vi "UMLEditor Main.vi"(1 "StartProject":string, 3 "StartTarget":string) -> ()   [LabVIEW 2012] (continued)
        n121 = call <resource>:"UMLEditor getDiagramInfo.vi"("localVariables"=w272, "error in (no error)"=w281) -> ("graph"=w279:refnum<class "Graph.lvclass">, "diagramType"=w275:T11, "error out"=w280:errorcluster)  [unwired: 15 out]
        n122 = event shown="[0] \"Picture\": Mouse Down" {
          selector: w273 -> [_ _ _ _ _ _ _ _ _ _ _ _ _ _ _ _ _ _ _ _ _ _ _ _ _ _ _ _ _ _ _ _ _ _ _ _ _ _ _ _ _ _ _ _ _ _ _ _ _ _ _ _ _ _ _ _ _]
          dyn-events: _ -> [_ _ _ _ _ _ _ _ _ _ _ _ _ _ _ _ _ _ _ _ _ _ _ _ _ _ _ _ _ _ _ _ _ _ _ _ _ _ _ _ _ _ _ _ _ _ _ _ _ _ _ _ _ _ _ _ _]
          timeout: 10 ("t") -> [_ _ _ _ _ _ _ _ _ _ _ _ _ _ _ _ _ _ _ _ _ _ _ _ _ _ _ _ _ _ _ _ _ _ _ _ _ _ _ _ _ _ _ _ _ _ _ _ _ _ _ _ _ _ _ _ _]
          tunnel: w283 -> [w289 _ _ _ _ _ _ _ _ _ w1719 _ _ _ _ _ _ _ _ _ _ _ _ _ _ _ _ _ _ _ _ _ _ _ _ _ _ _ _ _ _ _ _ _ _ _ _ _ _ _ _ _ _ _ _ _ _]
          tunnel: w277 -> [w284 w858 w1039 w1164 w1250 w1263 w1313 w1351 w1387 w1412 w1718 w2326 w2430 w2718 w2723 w2726 w3208 w3213 w3256 w3279 w3305 w3313 w3317 w3320 w3331 w3342 w3354 w3369 w3379 w3391 w3401 w3412 w3423 w3434 w3446 w3456 w3468 w3479 w3490 w3501 w3512 w3523 w3534 w3545 w3556 w3567 w3577 w3588 w3599 w3610 w3621 w3632 w3644 w3663 w3694 w3754 w3797]
          tunnel: [w295 w857 w1038 w1179 w1250 w1272 w1314 w1352 w1388 w1432 w1714 w2325 w2443 w2719 w2724 w2728 w3209 w3214 w3257 w3274 w3304 w3314 w3317 w3320 w3331 w3342 w3354 w3369 w3379 w3391 w3401 w3412 w3423 w3434 w3446 w3456 w3468 w3479 w3490 w3501 w3512 w3523 w3534 w3545 w3556 w3567 w3577 w3588 w3599 w3610 w3621 w3632 w3644 w3663 w3694 w3753 w3797] -> w278
          tunnel: w280 -> [w293 w862 w1042 w1185 w1251 w1262 w1312 w1350 w1386 w1428 w1717 w2324 w2439 w2715 w2721 w2732 w3207 w3215 w3249 w3276 w3306 w3315 w3319 w3324 w3333 w3344 w3356 w3373 w3384 w3395 w3406 w3417 w3428 w3439 w3450 w3461 w3472 w3483 w3494 w3505 w3516 w3527 w3538 w3549 w3560 w3571 w3582 w3589 w3600 w3611 w3622 w3633 w3646 w3656 w3692 w3750 w3802]
          tunnel: [w292 w864 w1044 w1174 w1251 w1262 w1312 w1350 w1386 w1423 w1716 w2323 w2440 w2715 w2721 w2731 w3207 w3215 w3249 w3260 w3306 w3315 w3319 w3323 w3332 w3343 w3355 w3372 w3383 w3394 w3405 w3416 w3427 w3438 w3449 w3460 w3471 w3482 w3493 w3504 w3515 w3526 w3537 w3548 w3559 w3570 w3581 w3590 w3601 w3612 w3623 w3634 w3645 w3657 w3695 w3755 w3801] -> w282
          tunnel: w279 -> [w296 w855 w1036 w1170 _ _ _ _ _ w1424 w1715 _ w2438 _ _ w2730 _ _ _ _ _ _ _ _ _ _ _ _ _ _ _ _ _ _ _ _ _ _ _ _ _ _ _ _ _ _ _ _ _ _ _ _ _ _ _ w3752 _]
          tunnel: w275 -> [w294 _ _ _ _ _ _ _ _ _ _ _ w2437 _ _ w2729 _ _ _ _ _ _ _ _ _ _ w3350 _ _ _ _ _ _ _ _ _ _ _ _ _ _ _ _ _ _ _ _ _ _ _ _ _ _ _ _ _ _]
          tunnel: w272 -> [_ w854 _ _ _ _ _ _ _ _ _ _ _ _ _ w2727 _ _ _ _ _ _ _ _ _ _ _ _ _ _ _ _ _ _ _ _ _ _ _ _ _ _ _ _ _ _ _ _ _ _ _ _ _ _ _ _ _]
          tunnel: w271 -> [w285 _ _ _ _ _ _ _ _ w1401 w1713 _ _ _ _ _ _ _ _ _ _ w3307 w3316 _ _ _ _ _ _ _ _ _ _ _ _ _ _ _ _ _ _ _ _ _ _ _ _ _ _ _ _ _ _ _ _ _ _]
          event "Picture": Mouse Down {
            # "Shift"
            n123 = event-data() -> ("Source"=w297:T41, "Button"=w291:u16, "Mods.Double Click"=w288:bool, "PlatMods.Ctrl"=w287:bool, "PlatMods.Shift"=w286:bool)  [unwired: 1 out]
            n124 = case shown="1, Default" w291 {
              tunnel: w297 -> [_ _]
              tunnel: w296 -> [w304 _]
              tunnel: [w339 w851] -> w295
              tunnel: w294 -> [w338 _]
              tunnel: w293 -> [w331 w850]
              tunnel: w284 -> [w324 w851]
              tunnel: [w326 w850] -> w292
              tunnel: w291 -> [w325 _]
              tunnel: w288 -> [w314 _]
              tunnel: w287 -> [w313 _]
              tunnel: w289 -> [_ _]
              tunnel: w286 -> [w303 _]
              tunnel: w285 -> [w299 _]
              frame 1, Default {
                n125 = property on="Picture" class="Pict"() -> ("Mouse"=w318:T42, "Draw Area Size"=w317:T43, "Origin"=w315:T44)  [unwired: 2 in, 2 out]
                n126 = Unbundle By Name(w324) -> ("graphics"=w307:refnum<class "Graphics.lvclass">, "SelectedNodes"=w320:refnum<class "AbstractNode.lvclass">[])
                n127 = Unbundle By Name(w324) -> ("HotSpotNode"=w300:refnum<class "AbstractNode.lvclass">, "HotSpotCursor"=w301:bool, "HotSpotFunction"=w302:T19, "zoom"=w327:dbl, "offset"=w329:T12)
                n128 = Unbundle By Name(w318) -> ("Mouse Position"=w330:cluster{"X":i32, "Y":i32})
                n129 = call <resource>:"UMLEditor ToolBarSettings.vi"("localVariables"=w324, "error in (no error)"=w331) -> ("toolType"=w337:T9, "tools"=w336:T10, "prototypeEdge"=w335:refnum<class "AbstractEdge.lvclass">, "prototypeNode"=w334:refnum<class "AbstractNode.lvclass">, "error out"=w312:errorcluster)  [unwired: 2 in, 11 out]
                n130 = Array Size(array=w320) -> (size(s)=w322:i32)
                n131 = Tick Count (ms)() -> (millisecond timer value=w319:u32)
                n132 = Greater?(x=w322, y=1) -> (0:w323:bool)
                n133 = Add(x=w329, y=w330) -> (x+y=w328:T12)
                n134 = call <resource>:"UMLEditor IsMouseOutsideDrawingArea.vi"("Mouse"=w318, "Draw Area Size"=w317, "Origin"=w315) -> ("OutsideDrawingArea"=w316:bool)  [unwired: 2 in, 14 out]
                n135 = Divide(x=w328, y=w327) -> (x/y=w311:T12)
                n136 = Bundle By Name(cluster=w324, "state"=UMLEditor_statesType."Repaint", "lastMousePoint"=w311) -> (w333:T7)
                n137 = call <resource>:"UMLEditor_FindObject.vi"("offset"=w311, "error in"=w312, "graphics"=w307, "graph"=w304) -> ("error out"=w310:errorcluster, "NodeFound"=w309:bool, "node"=w308:refnum<class "AbstractNode.lvclass">, "edge"=w306:refnum<class "AbstractEdge.lvclass">, "EdgeFound"=w305:bool)  [unwired: 2 in, 1 out]
                n138 = case shown="False" w316 {
                  tunnel: w310 -> [w372 w849]
                  tunnel: w309 -> [w345 _]
                  tunnel: w305 -> [w354 _]
                  tunnel: w306 -> [w371 _]
                  tunnel: w308 -> [w370 _]
                  tunnel: [w369 w847] -> w339
                  tunnel: w338 -> [w367 _]
                  tunnel: w337 -> [w366 _]
                  tunnel: w336 -> [w365 _]
                  tunnel: w335 -> [w364 _]
                  tunnel: w334 -> [w363 _]
                  tunnel: w304 -> [w362 _]
                  tunnel: w333 -> [w361 w848]
                  tunnel: w311 -> [w360 _]
                  tunnel: [w359 w849] -> w326
                  tunnel: w325 -> [w358 _]
                  tunnel: w323 -> [w357 _]
                  tunnel: w320 -> [w356 _]
                  tunnel: w319 -> [_ _]
                  tunnel: w317 -> [_ _]
                  tunnel: w314 -> [w346 _]
                  tunnel: w313 -> [w351 _]
                  tunnel: w307 -> [w349 _]
                  tunnel: w303 -> [w344 _]
                  tunnel: w302 -> [_ _]
                  tunnel: w301 -> [w342 _]
                  tunnel: w300 -> [w341 _]
                  tunnel: w299 -> [w340 _]
                  frame False {
                    n139 = Or(x=w345, y=w354) -> (x .or. y?=w353:bool)
                    n140 = And(x=w345, y=w344) -> (x .and. y?=w343:bool)
                    n141 = Compound Arithmetic op=AND(w346, w353) -> (w355:bool)
                    n142 = case shown="False" w355 {
                      tunnel: w372 -> [w392 w798]
                      tunnel: [w391 w797] -> w359
                      tunnel: w345 -> [w394 w796]
                      tunnel: w354 -> [w382 w791]
                      tunnel: w366 -> [w381 _]
                      tunnel: w361 -> [w397 w795]
                      tunnel: [w396 w794] -> w368
                      tunnel: w371 -> [w395 w793]
                      tunnel: w370 -> [w393 w792]
                      tunnel: w360 -> [w390 w789]
                      tunnel: w365 -> [w389 _]
                      tunnel: w367 -> [w388 _]
                      tunnel: w364 -> [w387 _]
                      tunnel: w363 -> [w386 _]
                      tunnel: w362 -> [w385 _]
                      tunnel: w358 -> [_ _]
                      tunnel: w357 -> [w384 _]
                      tunnel: w356 -> [w383 _]
                      tunnel: UMLEditor_tooltype."None" ("t") -> [w380 _]
                      tunnel: w351 -> [w377 w790]
                      tunnel: [TRUE ("butDwn") w788] -> w350
                      tunnel: w349 -> [w378 _]
                      tunnel: w343 -> [w376 _]
                      tunnel: [w376 w788] -> w348
                      tunnel: [w377 w788] -> w347
                      tunnel: w346 -> [_ _]
                      tunnel: w342 -> [w375 _]
                      tunnel: w341 -> [w374 _]
                      tunnel: w340 -> [w373 _]
                      frame False {
                        # "Single Click"
                        n143 = case shown="False" w376 {
                          tunnel: w397 -> [w420 w776]
                          tunnel: [w419 w775] -> w396
                          tunnel: w395 -> [w418 _]
                          tunnel: w394 -> [w417 _]
                          tunnel: w393 -> [w416 w772]
                          tunnel: w392 -> [w415 w771]
                          tunnel: [w414 w771] -> w391
                          tunnel: w390 -> [w413 w774]
                          tunnel: w389 -> [w412 _]
                          tunnel: w388 -> [w411 _]
                          tunnel: w387 -> [w410 _]
                          tunnel: w386 -> [w409 _]
                          tunnel: w385 -> [w408 _]
                          tunnel: w384 -> [w407 _]
                          tunnel: w383 -> [w406 w773]
                          tunnel: w382 -> [w405 _]
                          tunnel: w381 -> [w404 _]
                          tunnel: w380 -> [w402 _]
                          tunnel: w378 -> [w401 _]
                          tunnel: [_ w769] -> _
                          tunnel: w375 -> [w400 _]
                          tunnel: w374 -> [w399 _]
                          tunnel: w373 -> [w398 _]
                          frame False {
                            n144 = Select(t=w402, s=w405, f=w404) -> (s? t:f=w403:T9)
                            n145 = case shown="False" w400 {
                              tunnel: w420 -> [w440 w761]
                              tunnel: [w439 w760] -> w419
                              tunnel: w418 -> [w438 _]
                              tunnel: w417 -> [w437 _]
                              tunnel: w416 -> [w436 _]
                              tunnel: w415 -> [w435 w763]
                              tunnel: [w434 w762] -> w414
                              tunnel: w413 -> [w433 w759]
                              tunnel: w412 -> [w432 _]
                              tunnel: w411 -> [w431 _]
                              tunnel: w410 -> [w430 _]
                              tunnel: w409 -> [w429 _]
                              tunnel: w408 -> [w428 _]
                              tunnel: w407 -> [w427 _]
                              tunnel: w406 -> [w426 _]
                              tunnel: w405 -> [w425 _]
                              tunnel: w403 -> [w424 _]
                              tunnel: w401 -> [w423 _]
                              tunnel: w400 -> [w422 _]
                              tunnel: w399 -> [_ w758]
                              tunnel: w398 -> [w421 _]
                              frame False {
                                n146 = case shown="\"Node\"" w424 {
                                tunnel: w425 -> [w455 _ _]
                                tunnel: w440 -> [w454 w591 w640]
                                tunnel: [w453 w590 w639] -> w439
                                tunnel: w438 -> [w452 _ _]
                                tunnel: w437 -> [w451 w586 w637]
                                tunnel: w436 -> [w450 w585 w636]
                                tunnel: w435 -> [w449 w583 w635]
                                tunnel: [w448 w587 w634] -> w434
                                tunnel: w433 -> [w447 w582 w638]
                                tunnel: w432 -> [_ _ w633]
                                tunnel: w431 -> [_ _ w632]
                                tunnel: w430 -> [_ _ _]
                                tunnel: w429 -> [_ w594 _]
                                tunnel: w428 -> [w446 w584 w631]
                                tunnel: w427 -> [w445 _ _]
                                tunnel: w426 -> [w444 _ _]
                                tunnel: w423 -> [w443 _ _]
                                tunnel: w422 -> [w442 _ _]
                                tunnel: w421 -> [w441 _ _]
                                frame "None", Default {
                                # "Select"
                                n147 = case shown="False" w455 {
                                tunnel: w454 -> [w465 w560]
                                tunnel: [w464 w559] -> w453
                                tunnel: w452 -> [_ w523]
                                tunnel: w451 -> [w466 _]
                                tunnel: w450 -> [w463 _]
                                tunnel: w449 -> [w462 w539]
                                tunnel: [w461 w539] -> w448
                                tunnel: w447 -> [w460 w534]
                                tunnel: w446 -> [_ _]
                                tunnel: w445 -> [w459 _]
                                tunnel: w444 -> [w458 _]
                                tunnel: w443 -> [_ w520]
                                tunnel: w442 -> [w457 _]
                                tunnel: w441 -> [w456 _]
                                frame False {
                                n148 = case shown="True" w466 {
                                tunnel: w465 -> [w471 w518]
                                tunnel: [w476 w517] -> w464
                                tunnel: w463 -> [w477 _]
                                tunnel: w462 -> [w478 w514]
                                tunnel: [w475 w514] -> w461
                                tunnel: w460 -> [w474 w511]
                                tunnel: w459 -> [w473 _]
                                tunnel: w458 -> [w472 _]
                                tunnel: w457 -> [w468 _]
                                tunnel: w456 -> [w467 _]
                                frame True {
                                # "Node Selected"
                                n149 = case shown="False" w468 {
                                tunnel: w467 -> [w479 _]
                                frame False {
                                n150 = call-poly <vilib>:"Set Cursor.vi"("VI reference (current VI)"=w479, "icon"=u16 5) -> ()  [unwired: 1 in, 9 out]
                                }
                                frame True {
                                }
                                }
                                n151 = Bundle By Name(cluster=w471, "state"=UMLEditor_statesType."Idle") -> (w469:T7)
                                n152 = case shown="True" w473 {
                                tunnel: w478 -> [w490 w494]
                                tunnel: w477 -> [w489 w493]
                                tunnel: w469 -> [w486 w492]
                                tunnel: [w485 w498] -> w476
                                tunnel: [w483 w494] -> w475
                                tunnel: w474 -> [w481 w497]
                                tunnel: w472 -> [_ w496]
                                frame False {
                                n153 = call-dynamic "getBounds.vi"("reference"=w489, "error in (no error)"=w490) -> ("reference out"=w488:refnum<class "AbstractNode.lvclass">, "bounds"=w487:T13, "error out"=w483:errorcluster)  [unwired: 15 in]
                                n154 = Build Array(w488) -> (w482:refnum<class "AbstractNode.lvclass">[])
                                n155 = Bundle By Name(cluster=w486, "selcted"=UMLEditor_tooltype."Node", "SelectedNodes"=w482, "dragStartBounds"=w487, "dragStartPoint"=w481, "newSelected"=TRUE, "lastMousePoint"=w481) -> (w485:T7)
                                }
                                frame True {
                                # "If many nodes allready selected move these"
                                n156 = Search 1D Array(1D array=w496, element=w493) -> (index of element=w495:i32)  [unwired: 1 out]
                                n157 = case shown="Default" w495 {
                                tunnel: w492 -> [w503 w510]
                                tunnel: [w502 w509] -> w498
                                tunnel: w497 -> [w501 w508]
                                tunnel: w493 -> [_ w505]
                                frame Default {
                                n158 = Bundle By Name(cluster=w503, "selcted"=UMLEditor_tooltype."Node", "dragStartPoint"=w501, "newSelected"=TRUE, "lastMousePoint"=w501) -> (w502:T7)
                                }
                                frame -1 {
                                n159 = Build Array(w505) -> (w504:refnum<class "AbstractNode.lvclass">[])
                                n160 = Bundle By Name(cluster=w510, "selcted"=UMLEditor_tooltype."Node", "dragStartPoint"=w508, "newSelected"=TRUE, "lastMousePoint"=w508, "SelectedNodes"=w504) -> (w509:T7)
                                }
                                }
                                }
                                }
                                }
                                frame False {
                                # "None Selected\nArea Select???"
                                n161 = Bundle By Name(cluster=w518, "selcted"=UMLEditor_tooltype."None", "SelectedNodes"=refnum<class "AbstractNode.lvclass">[] [], "dragStartBounds"=T13 {"x"=0.0, "y"=0.0, "width"=0.0, "height"=0.0}, "dragStartPoint"=w511, "rubberBandStart"=w511, "newSelected"=TRUE, "state"=UMLEditor_statesType."Idle", "lastMousePoint"=w511) -> (w517:T7)
                                }
                                }
                                }
                                frame True {
                                w556 = 25.0 ("y")
                                n162 = To More Specific Class(target class=refnum<class "GeneralPathEdge.lvclass"> refnum ("reference"), reference=w523) -> (specific class reference=w521:refnum<class "GeneralPathEdge.lvclass">)  [unwired: 1 in, 1 out]
                                n163 = call-dynamic "getPoints.vi"("reference"=w521, "error in (no error)"=w539) -> ("reference out"=w537:refnum<class "GeneralPathEdge.lvclass">, "points"=w535:T12[], "error out"=w538:errorcluster)  [unwired: 15 in]
                                n164 = Array Size(array=w535) -> (size(s)=w536:i32)
                                n165 = case shown="4" w536 {
                                tunnel: w535 -> [_ w569]
                                tunnel: w534 -> [_ w564]
                                tunnel: [_ w561] -> w529
                                frame Default {
                                }
                                frame 4 {
                                # "Egde selected"
                                n166 = Index Array(array=w569, index #1=1 ("index")) -> (element #1=w567:T12, element #2=w566:T12)  [unwired: 1 in]
                                n167 = Build Array(w567, w566) -> (w565:T12[])
                                n168 = call <resource>:"Point getDistanceToLine.vi"("point1"=w564, "line"=w565) -> ("minDistance"=w563:dbl)  [unwired: 1 in, 16 out]
                                n169 = Less?(x=w563, y=25.0) -> (x < y?=w561:bool)
                                }
                                }
                                n170 = Index Array(array=w535) -> (element=w555:T12)  [unwired: 1 in]
                                n171 = Delete From Array(array=w535) -> (deleted portion=w554:T12)  [unwired: 2 in, 1 out]
                                n172 = call-dynamic "GetTextPositions.vi"("reference"=w537, "GraphicsRef"=w520, "error in (no error)"=w538) -> ("reference out"=w547:refnum<class "GeneralPathEdge.lvclass">, "connectionPoints"=w546:T12[], "error out"=w548:errorcluster)  [unwired: 14 in]
                                n173 = Index Array(array=w546) -> (element=w545:T12)  [unwired: 1 in]
                                n174 = call <resource>:"Point getDistance.vi"("point1"=w555, "point2"=w534) -> ("distance"=w558:dbl)  [unwired: 1 in, 16 out]
                                n175 = call <resource>:"Point getDistance.vi"("point1"=w554, "point2"=w534) -> ("distance"=w557:dbl)  [unwired: 1 in, 16 out]
                                n176 = call-dynamic "getEnd.vi"("reference"=w547, "error in (no error)"=w548) -> ("reference out"=w552:refnum<class "GeneralPathEdge.lvclass">, "endNode"=w526:refnum<class "AbstractNode.lvclass">, "error out"=w553:errorcluster)  [unwired: 14 in, 1 out]
                                n177 = call <resource>:"Point getDistance.vi"("point1"=w545, "point2"=w534) -> ("distance"=w544:dbl)  [unwired: 1 in, 16 out]
                                n178 = Less?(x=w557, y=w556) -> (x < y?=w532:bool)
                                n179 = Less?(x=w558, y=w556) -> (x < y?=w531:bool)
                                n180 = Less?(x=w544, y=40.0) -> (x < y?=w533:bool)
                                n181 = call-dynamic "getStart.vi"("reference"=w552, "error in (no error)"=w553) -> ("startNode"=w525:refnum<class "AbstractNode.lvclass">, "error out"=w551:errorcluster)  [unwired: 14 in, 2 out]
                                n182 = Select(t=w526, s=w532, f=w525) -> (s? t:f=w542:refnum<class "AbstractNode.lvclass">)
                                n183 = Unbundle By Name(w551) -> ("status"=w550:bool)
                                n184 = Build Array(w526, w525) -> (w524:refnum<class "AbstractNode.lvclass">[])
                                n185 = Compound Arithmetic op=OR(w529, w531, w532, w533) -> (w530:bool)
                                n186 = Build Array(w542) -> (w528:refnum<class "AbstractNode.lvclass">[])
                                n187 = Compound Arithmetic op=AND(w530, invert w550) -> (w549:bool)
                                n188 = Select(t=w524, s=w529, f=w528) -> (s? t:f=w527:refnum<class "AbstractNode.lvclass">[])
                                n189 = Select(t=refnum<class "AbstractNode.lvclass">[] [], s=w533, f=w527) -> (s? t:f=w540:refnum<class "AbstractNode.lvclass">[])
                                n190 = case shown="True" w549 {
                                tunnel: w560 -> [w576 w581]
                                tunnel: [w575 w580] -> w559
                                tunnel: w523 -> [w572 w577]
                                tunnel: w534 -> [w571 _]
                                tunnel: w540 -> [w570 _]
                                frame True {
                                n191 = Bundle By Name(cluster=w576, "selcted"=UMLEditor_tooltype."Edge", "selectedEdge"=w572, "dragStartPoint"=w571, "newSelected"=TRUE, "SelectedNodes"=w570) -> (w575:T7)
                                }
                                frame False {
                                n192 = Bundle By Name(cluster=w581, "selcted"=UMLEditor_tooltype."Edge", "selectedEdge"=w577, "newSelected"=TRUE) -> (w580:T7)
                                }
                                }
                                }
                                }
                                }
                                frame "Node" {
                                # "Node Tool"
                                n193 = call-dynamic "clone.vi"("reference"=w594, "error in (no error)"=w583) -> ("clonedAbstractNode"=w588:refnum<class "AbstractNode.lvclass">, "error out"=w593:errorcluster)  [unwired: 15 in, 1 out]
                                n194 = call-dynamic "add.vi"("reference"=w584, "node"=w588, "point"=w582, "error in (no error)"=w593) -> ("added"=w592:bool, "error out"=w589:errorcluster)  [unwired: 13 in, 1 out]
                                n195 = case shown="False" w592 {
                                tunnel: w591 -> [w602 w622]
                                tunnel: [w601 w620] -> w590
                                tunnel: w589 -> [w597 w630]
                                tunnel: w588 -> [w595 w629]
                                tunnel: w582 -> [w599 w618]
                                tunnel: [w598 w623] -> w587
                                tunnel: w586 -> [w603 _]
                                tunnel: w585 -> [w600 _]
                                frame False {
                                n196 = call-dynamic "Destroy.vi"("reference"=w595, "error in (no error)"=w597) -> ("error out"=w596:errorcluster)  [unwired: 16 in, 1 out]
                                n197 = case shown="False" w603 {
                                tunnel: w602 -> [w605 w614]
                                tunnel: [w605 w613] -> w601
                                tunnel: w596 -> [w604 w616]
                                tunnel: w600 -> [_ w608]
                                tunnel: w599 -> [_ w610]
                                tunnel: [w604 w612] -> w598
                                frame False {
                                }
                                frame True {
                                # "Node Found"
                                n198 = call-dynamic "getBounds.vi"("reference"=w608, "error in (no error)"=w616) -> ("bounds"=w615:T13, "error out"=w612:errorcluster)  [unwired: 15 in, 1 out]
                                n199 = Build Array(w608) -> (w611:refnum<class "AbstractNode.lvclass">[])
                                n200 = Bundle By Name(cluster=w614, "selcted"=UMLEditor_tooltype."Node", "SelectedNodes"=w611, "dragStartBounds"=w615, "dragStartPoint"=w610, "lastMousePoint"=w610, "newSelected"=TRUE, "toolType"=UMLEditor_tooltype."None", "tool"=UMLEditor_toolsType."CD_Select") -> (w613:T7)
                                n201 = call <resource>:"UMLEditor UpdatesToolbuttons.vi"() -> ()  [unwired: 6 in, 14 out]
                                }
                                }
                                }
                                frame True {
                                # "Added"
                                n202 = call-dynamic "getBounds.vi"("reference"=w629, "error in (no error)"=w630) -> ("reference out"=w627:refnum<class "AbstractNode.lvclass">, "bounds"=w628:T13, "error out"=w624:errorcluster)  [unwired: 15 in]
                                n203 = Build Array(w627) -> (w619:refnum<class "AbstractNode.lvclass">[])
                                n204 = Bundle By Name(cluster=w622, "selcted"=UMLEditor_tooltype."Node", "SelectedNodes"=w619, "dragStartBounds"=w628, "dragStartPoint"=w618, "lastMousePoint"=w618) -> (w621:T7)
                                n205 = call <resource>:"UMLEditor setDiagramInfo.vi"("error in (no error)"=w624, "localVariablesIn"=w621, "action"=enum16{"Name/Dir", "Unsaved", "Saved"}."Unsaved") -> ("localVariablesOut"=w620:T7, "error out"=w623:errorcluster)  [unwired: 2 in, 13 out]
                                }
                                }
                                }
                                frame "Edge" {
                                # "Edge Tool"
                                n206 = case shown="True" w637 {
                                tunnel: w640 -> [w642 w655]
                                tunnel: [w641 w654] -> w639
                                tunnel: w638 -> [_ w653]
                                tunnel: w636 -> [_ w652]
                                tunnel: w635 -> [w645 w651]
                                tunnel: [w645 w649] -> w634
                                tunnel: w633 -> [_ w648]
                                tunnel: w632 -> [_ w647]
                                tunnel: w631 -> [_ w646]
                                frame False {
                                n207 = call <resource>:"UMLEditor UpdatesToolbuttons.vi"() -> ()  [unwired: 6 in, 14 out]
                                n208 = Bundle By Name(cluster=w642, "toolType"=UMLEditor_tooltype."None", "tool"=UMLEditor_toolsType."CD_Select") -> (w641:T7)
                                }
                                frame True {
                                n209 = case shown="\"Class\"" w647 {
                                tunnel: w652 -> [_ w685 w698 w711 w743]
                                tunnel: w651 -> [w656 w684 w699 w712 w742]
                                tunnel: [TRUE w668 w695 w707 w727] -> w650
                                tunnel: [w656 w667 w697 w710 w734] -> w649
                                tunnel: w648 -> [_ w665 w686 w706 w720]
                                tunnel: w646 -> [_ _ _ _ w736]
                                frame "None", Default {
                                }
                                frame "Class" {
                                w664 = UMLEditor_toolsType."CD_Dependency" ("tools")
                                n210 = call <resource>:"AbstractNode_GetObjectStatus.vi"("reference in"=w685, "error in (no error)"=w684) -> ("Class name"=w659:string, "error out"=w667:errorcluster)  [unwired: 16 out]
                                n211 = Match Pattern(string=w659, regular expression="NoteNode$") -> (offset past match=w680:i32)  [unwired: 4 out]
                                n212 = Match Pattern(string=w659, regular expression="InterfaceNode$") -> (offset past match=w679:i32)  [unwired: 4 out]
                                n213 = Match Pattern(string=w659, regular expression="ClassNode$") -> (offset past match=w678:i32)  [unwired: 4 out]
                                n214 = Match Pattern(string=w659, regular expression="PackageNode$") -> (offset past match=w661:i32)  [unwired: 4 out]
                                n215 = Equal?(x=w665, y=UMLEditor_toolsType."CD_NoteConn" ("tools")) -> (x = y?=w672:bool)
                                n216 = In Range and Coerce(upper limit=UMLEditor_toolsType."CD_Composite" ("tools"), x=w665, lower limit=w664) -> (In Range?=w675:bool)  [unwired: 1 out]
                                n217 = Equal?(x=w664, y=w665) -> (x = y?=w662:bool)
                                n218 = Greater Or Equal To 0?(x=w680) -> (x >= 0?=w671:bool)
                                n219 = Greater Or Equal To 0?(x=w679) -> (x >= 0?=w677:bool)
                                n220 = Greater Or Equal To 0?(x=w678) -> (x >= 0?=w676:bool)
                                n221 = Greater Or Equal To 0?(x=w661) -> (x >= 0?=w658:bool)
                                n222 = And(x=w672, y=w671) -> (x .and. y?=w669:bool)
                                n223 = Or(x=w677, y=w676) -> (x .or. y?=w674:bool)
                                n224 = And(x=w675, y=w674) -> (x .and. y?=w670:bool)
                                n225 = And(x=w662, y=w658) -> (x .and. y?=w663:bool)
                                n226 = Compound Arithmetic op=OR(w670, w669, w663) -> (w668:bool)
                                }
                                frame "Sequency" {
                                n227 = call <resource>:"AbstractNode_GetObjectStatus.vi"("reference in"=w698, "error in (no error)"=w699) -> ("Class name"=w688:string, "error out"=w697:errorcluster)  [unwired: 16 out]
                                n228 = Match Pattern(string=w688, regular expression="CallNode$") -> (offset past match=w690:i32)  [unwired: 4 out]
                                n229 = Match Pattern(string=w688, regular expression="NoteNode$") -> (offset past match=w702:i32)  [unwired: 4 out]
                                n230 = Equal?(x=w686, y=UMLEditor_toolsType."SQD_Call" ("tools")) -> (x = y?=w691:bool)
                                n231 = Equal?(x=w686, y=UMLEditor_toolsType."SQD_NoteConn" ("tools")) -> (x = y?=w701:bool)
                                n232 = Greater Or Equal To 0?(x=w690) -> (x >= 0?=w692:bool)
                                n233 = Greater Or Equal To 0?(x=w702) -> (x >= 0?=w700:bool)
                                n234 = And(x=w691, y=w692) -> (x .and. y?=w687:bool)
                                n235 = And(x=w701, y=w700) -> (x .and. y?=w696:bool)
                                n236 = Compound Arithmetic op=OR(w687, w696) -> (w695:bool)
                                }
                                frame "UseCase" {
                                w705 = UMLEditor_toolsType."UD_NoteEdge" ("tools")
                                n237 = call <resource>:"AbstractNode_GetObjectStatus.vi"("reference in"=w711, "error in (no error)"=w712) -> ("Class name"=w709:string, "error out"=w710:errorcluster)  [unwired: 16 out]
                                n238 = Not Equal?(x=w706, y=w705) -> ()  [unwired: 1 out]
                                n239 = Match Pattern(string=w709, regular expression="NoteNode$") -> (offset past match=w714:i32)  [unwired: 4 out]
                                n240 = Equal?(x=w706, y=w705) -> (x = y?=w713:bool)
                                n241 = Greater Or Equal To 0?(x=w714) -> (x >= 0?=w704:bool)
                                n242 = And(x=w713, y=w704) -> (x .and. y?=w708:bool)
                                n243 = Compound Arithmetic op=OR(invert w704, w708) -> (w707:bool)
                                }
                                frame "State" {
                                w735 = "InitialStateNode$" ("regular expression")
                                n244 = call <resource>:"AbstractNode_GetObjectStatus.vi"("reference in"=w743, "error in (no error)"=w742) -> ("Class name"=w722:string, "error out"=w737:errorcluster)  [unwired: 16 out]
                                n245 = call-dynamic "getEdges.vi"("reference"=w736, "error in (no error)"=w737) -> ("edges"=w733:refnum<class "AbstractEdge.lvclass">[], "error out"=w734:errorcluster)  [unwired: 15 in, 1 out]
                                n246 = for {
                                tunnel: w734 -> [w751]
                                tunnel: w735 -> [w750]
                                tunnel: [w748] -> w732 mode=indexing
                                tunnel: w733 -> [w747] mode=indexing
                                n247 = call-dynamic "getStart.vi"("reference"=w747, "error in (no error)"=w751) -> ("startNode"=w746:refnum<class "AbstractNode.lvclass">, "error out"=w745:errorcluster)  [unwired: 14 in, 2 out]
                                n248 = call <resource>:"AbstractNode_GetObjectStatus.vi"("reference in"=w746, "error in (no error)"=w745) -> ("Class name"=w744:string)  [unwired: 17 out]
                                n249 = Match Pattern(string=w744, regular expression=w750) -> (offset past match=w749:i32)  [unwired: 4 out]
                                n250 = Greater Or Equal To 0?(x=w749) -> (x >= 0?=w748:bool)
                                }
                                n251 = Match Pattern(string=w722, regular expression="FinalStateNode$") -> (offset past match=w740:i32)  [unwired: 4 out]
                                n252 = Match Pattern(string=w722, regular expression="NoteNode$") -> (offset past match=w725:i32)  [unwired: 4 out]
                                n253 = Match Pattern(string=w722, regular expression=w735) -> (offset past match=w739:i32)  [unwired: 4 out]
                                n254 = Equal?(x=w720, y=UMLEditor_toolsType."STD_NoteEdge" ("tools")) -> (x = y?=w724:bool)
                                n255 = Equal?(x=w720, y=UMLEditor_toolsType."STD_StateTransation" ("tools")) -> (x = y?=w717:bool)
                                n256 = Greater Or Equal To 0?(x=w725) -> (x >= 0?=w718:bool)
                                n257 = Greater Or Equal To 0?(x=w740) -> (x >= 0?=w738:bool)
                                n258 = Greater Or Equal To 0?(x=w739) -> (x >= 0?=w731:bool)
                                n259 = Or Array Elements(Boolean array=w732) -> (logical OR=w730:bool)
                                n260 = And(x=w724, y=w718) -> (x .and. y?=w721:bool)
                                n261 = And(x=w718, y=w717) -> (x .and. y?=w716:bool)
                                n262 = And(x=w731, y=w730) -> (x .and. y?=w729:bool)
                                n263 = Compound Arithmetic op=OR(w716, w738, w729) -> (invert w728:bool)
                                n264 = Compound Arithmetic op=OR(w721, w728) -> (w727:bool)
                                }
                                }
                                n265 = case shown="True" w650 {
                                tunnel: w655 -> [w752 w757]
                                tunnel: [w752 w756] -> w654
                                tunnel: w653 -> [_ w755]
                                frame False {
                                }
                                frame True {
                                n266 = Bundle By Name(cluster=w757, "rubberBandStart"=w755, "selcted"=UMLEditor_tooltype."Edge", "state"=UMLEditor_statesType."Idle") -> (w756:T7)
                                }
                                }
                                }
                                }
                                }
                                }
                              }
                              frame True {
                                n267 = call-dynamic "getBounds.vi"("reference"=w758, "error in (no error)"=w763) -> ("reference out"=w767:refnum<class "AbstractNode.lvclass">, "bounds"=w766:T13, "error out"=w762:errorcluster)  [unwired: 15 in]
                                n268 = Build Array(w767) -> (w764:refnum<class "AbstractNode.lvclass">[])
                                n269 = Bundle By Name(cluster=w761, "selcted"=UMLEditor_tooltype."Node", "SelectedNodes"=w764, "dragStartBounds"=w766, "dragStartPoint"=w759, "newSelected"=TRUE, "lastMousePoint"=w759) -> (w760:T7)
                              }
                            }
                          }
                          frame True {
                            # "Shift Click"
                            n270 = Search 1D Array(1D array=w773, element=w772) -> (index of element=w781:i32)  [unwired: 1 in]
                            n271 = case shown="0, Default" w781 {
                              selector: w781 -> [w782 _]
                              tunnel: w773 -> [w784 w787]
                              tunnel: w772 -> [_ w786]
                              tunnel: [w783 w785] -> w770
                              frame 0, Default {
                                n272 = Delete From Array(array=w784, index=w782) -> (array with subset deleted=w783:refnum<class "AbstractNode.lvclass">[])  [unwired: 1 in, 1 out]
                              }
                              frame -1 {
                                n273 = Build Array (concatenate)(w787, w786) -> (w785:refnum<class "AbstractNode.lvclass">[])
                              }
                            }
                            n274 = Bundle By Name(cluster=w776, "selcted"=UMLEditor_tooltype."Node", "SelectedNodes"=w770, "dragStartBounds"=T13 {"x"=nan, "y"=nan, "width"=nan, "height"=nan}, "dragStartPoint"=T12 {"x"=nan, "y"=nan}, "newSelected"=TRUE, "lastMousePoint"=w774) -> (w775:T7)
                            n275 = Array Size(array=w770) -> (size(s)=w769:i32)
                          }
                        }
                      }
                      frame True {
                        w788 = FALSE ("butDwn")
                        # "DblClick"
                        n276 = case shown="False" w791 {
                          tunnel: w798 -> [w807 w841]
                          tunnel: [w806 w841] -> w797
                          tunnel: w796 -> [w805 _]
                          tunnel: w795 -> [w804 w843]
                          tunnel: [w803 w842] -> w794
                          tunnel: w793 -> [w802 w840]
                          tunnel: w792 -> [w801 _]
                          tunnel: w790 -> [w800 _]
                          tunnel: w789 -> [w799 _]
                          frame False {
                            n277 = case shown="True" w805 {
                              tunnel: w807 -> [w808 w813]
                              tunnel: [w808 w812] -> w806
                              tunnel: w804 -> [w809 w816]
                              tunnel: [w809 w815] -> w803
                              tunnel: w802 -> [_ _]
                              tunnel: w801 -> [_ w810]
                              tunnel: w800 -> [_ w814]
                              tunnel: w799 -> [_ w811]
                              frame False {
                              }
                              frame True {
                                # "Node Found"
                                n278 = case shown="True" w814 {
                                tunnel: w816 -> [w821 w828]
                                tunnel: [w820 w827] -> w815
                                tunnel: w810 -> [w818 _]
                                tunnel: w813 -> [w817 w832]
                                tunnel: [w817 w831] -> w812
                                tunnel: w811 -> [_ w830]
                                tunnel: w810 -> [_ w829]
                                frame False {
                                n279 = Build Array(w818) -> (w819:refnum<class "AbstractNode.lvclass">[])
                                n280 = Bundle By Name(cluster=w821, "selcted"=UMLEditor_tooltype."Node", "SelectedNodes"=w819, "state"=UMLEditor_statesType."EditSelected") -> (w820:T7)
                                }
                                frame True {
                                n281 = call-dynamic "GetContextHelpInfo.vi"("reference"=w829, "MousePos"=w830, "error in (no error)"=w832) -> ("ContextHelpInfo"=w826:variant, "error out"=w831:errorcluster)  [unwired: 13 in, 2 out]
                                n282 = Variant To Data(type=path "", Variant=w826) -> (error out=w824:errorcluster)  [unwired: 1 in, 1 out]
                                n283 = case shown="No Error" w824 {
                                tunnel: w828 -> [w837 w839]
                                tunnel: [w836 w839] -> w827
                                tunnel: w826 -> [w833 _]
                                frame No Error {
                                # "Ctrl-Key down\nSo lets open the method"
                                n284 = Bundle By Name(cluster=T15 {"Command"=enum."OpenFile", "CommandData"=variant} ("FlattenCommandSettings"), "CommandData"=w833) -> (w834:T15)
                                n285 = Bundle By Name(cluster=w837, "state"=UMLEditor_statesType."ExecuteCommand", "FlattenCommandSettings"=w834) -> (w836:T7)
                                }
                                frame Error {
                                }
                                }
                                }
                                }
                              }
                            }
                          }
                          frame True {
                            # "Edge Found"
                            n286 = Bundle By Name(cluster=w843, "selcted"=UMLEditor_tooltype."Edge", "selectedEdge"=w840, "state"=UMLEditor_statesType."EditSelected") -> (w842:T7)
                          }
                        }
                      }
                    }
                    n287 = Bundle By Name(cluster=w368, "butDwn"=w350, "ShiftDown"=w348, "CtrlDown"=w347) -> (w369:T7)
                  }
                  frame True {
                    # "SCROLLING"
                    n288 = Bundle By Name(cluster=w848, "state"=UMLEditor_statesType."Idle") -> (w847:T7)
                  }
                }
              }
              frame 0, 2 {
              }
            }
            n289 = property on="ClassAggregationDialog" class="Clust (strict)"() -> ("Visible"=w290:bool)  [unwired: 2 in, 2 out]
            n290 = case shown="False" w290 {
              frame False {
              }
              frame True {
                n291 = property on="ClassAggregationDialog" class="Clust (strict)"("Visible"=FALSE) -> ()  [unwired: 2 in, 2 out]
              }
            }
          }
          event "Picture": Shortcut Menu Selection (User) {
            n292 = event-data() -> ("ItemTag"=w859:string)  [unwired: 1 out]
            n293 = Unbundle By Name(w858) -> ("selcted"=w863:T9, "selectedEdge"=w856:refnum<class "AbstractEdge.lvclass">, "SelectedNodes"=w861:refnum<class "AbstractNode.lvclass">[])
            n294 = Unbundle By Name(w854) -> ("graphics"=w853:refnum<class "Graphics.lvclass">, "grid"=w852:refnum<class "Grid.lvclass">)
            n295 = Index Array(array=w861) -> (element=w860:refnum<class "AbstractNode.lvclass">)  [unwired: 1 in]
            n296 = case shown="\"Node\"" w863 {
              tunnel: [w871 w910 w954] -> w864
              tunnel: [w870 w906 w953] -> w857
              tunnel: w862 -> [w869 w909 w950]
              tunnel: w860 -> [_ _ w952]
              tunnel: w859 -> [w868 w907 w951]
              tunnel: w858 -> [w866 w905 w949]
              tunnel: w856 -> [w867 _ _]
              tunnel: w855 -> [w865 w908 w948]
              tunnel: w853 -> [_ _ w947]
              tunnel: w852 -> [_ _ w946]
              frame "Edge" {
                n297 = case shown="Default" w868 {
                  selector: w868 -> [w879 _ _]
                  tunnel: w869 -> [w881 w898 w902]
                  tunnel: w866 -> [w874 w900 w904]
                  tunnel: [w876 w897 w901] -> w870
                  tunnel: w867 -> [w880 _ _]
                  tunnel: [w875 w898 w902] -> w871
                  tunnel: w865 -> [w872 _ _]
                  frame Default {
                    n298 = call-dynamic "ExecuteMenuCommand.vi"("reference"=w880, "Command"=w879, "error in (no error)"=w881) -> ("reference out"=w877:refnum<class "AbstractEdge.lvclass">, "EditorAction"=w878:T45, "error out"=w873:errorcluster)  [unwired: 14 in]
                    n299 = case shown="\"ExecuteCommand\"" w878 {
                      tunnel: w874 -> [w882 w887 w896]
                      tunnel: [w882 w886 w893] -> w876
                      tunnel: w877 -> [_ _ _]
                      tunnel: w873 -> [w883 w891 w894]
                      tunnel: [w883 w889 w894] -> w875
                      tunnel: w872 -> [_ w885 _]
                      frame "NoAction", Default {
                      }
                      frame "Repaint" {
                        n300 = call-dynamic "layout.vi"("reference"=w885, "error in (no error)"=w891) -> ("error out"=w890:errorcluster)  [unwired: 16 in, 1 out]
                        n301 = Bundle By Name(cluster=w887, "state"=UMLEditor_statesType."Repaint") -> (w884:T7)
                        n302 = call <resource>:"UMLEditor setDiagramInfo.vi"("error in (no error)"=w890, "localVariablesIn"=w884, "action"=enum16{"Name/Dir", "Unsaved", "Saved"}."Unsaved") -> ("localVariablesOut"=w886:T7, "error out"=w889:errorcluster)  [unwired: 2 in, 13 out]
                      }
                      frame "ExecuteCommand" {
                        n303 = Bundle By Name(cluster=w896, "state"=UMLEditor_statesType."ExecuteCommand") -> (w893:T7)
                      }
                    }
                  }
                  frame "Remove Edge" {
                    n304 = Bundle By Name(cluster=w900, "state"=UMLEditor_statesType."RemoveSelected") -> (w897:T7)
                  }
                  frame "Configure Edge" {
                    n305 = Bundle By Name(cluster=w904, "state"=UMLEditor_statesType."EditSelected") -> (w901:T7)
                  }
                }
              }
              frame "None", Default {
                n306 = Unbundle By Name(w905) -> ("graphics"=w914:refnum<class "Graphics.lvclass">, "grid"=w913:refnum<class "Grid.lvclass">)
                n307 = Bundle By Name(cluster=w905, "state"=UMLEditor_statesType."Repaint") -> (w912:T7)
                n308 = case shown="\"Apply Design Pattern...\"" w907 {
                  selector: w907 -> [_ _ w931]
                  tunnel: w909 -> [w917 w918 w938]
                  tunnel: [w917 w918 w936] -> w911
                  tunnel: w914 -> [_ _ w930]
                  tunnel: w913 -> [_ _ w929]
                  tunnel: w912 -> [w916 w920 w935]
                  tunnel: [w916 w919 w934] -> w906
                  tunnel: w908 -> [_ _ w932]
                  tunnel: w905 -> [_ _ w922]
                  frame "" {
                  }
                  frame "Apply Design Pattern..." {
                    n309 = Bundle By Name(cluster=w920, "state"=UMLEditor_statesType."ApplyDesignPattern") -> (w919:T7)
                  }
                  frame Default {
                    n310 = property on="Picture" class="Pict"() -> ("Mouse"=w924:T42)  [unwired: 2 in, 2 out]
                    n311 = Unbundle By Name(w924) -> ("Mouse Position"=w928:cluster{"X":i32, "Y":i32})
                    n312 = Unbundle By Name(w922) -> ("zoom"=w925:dbl, "offset"=w927:T12)
                    n313 = Add(x=w927, y=w928) -> (x+y=w926:T12)
                    n314 = Divide(x=w926, y=w925) -> (x/y=w923:T12)
                    n315 = call-dynamic "HandleRightClickMenuOption.vi"("reference"=w932, "MenuOption"=w931, "graphics"=w930, "grid"=w929, "point2D"=w923, "error in (no error)"=w938) -> ("Cancel"=w933:bool, "error out"=w937:errorcluster)  [unwired: 11 in, 1 out]
                    n316 = case shown="False" w933 {
                      tunnel: w937 -> [w942 w945]
                      tunnel: [w941 w945] -> w936
                      tunnel: w935 -> [w939 w944]
                      tunnel: [w940 w944] -> w934
                      frame False {
                        n317 = call <resource>:"UMLEditor setDiagramInfo.vi"("error in (no error)"=w942, "localVariablesIn"=w939, "action"=enum16{"Name/Dir", "Unsaved", "Saved"}."Unsaved") -> ("localVariablesOut"=w940:T7, "error out"=w941:errorcluster)  [unwired: 2 in, 13 out]
                      }
                      frame True {
                      }
                    }
                  }
                }
                n318 = call <resource>:"UMLEditor UpdatesToolbuttons.vi"("error in (no error)"=w911) -> ("error out"=w910:errorcluster)  [unwired: 5 in, 13 out]
              }
              frame "Node" {
                n319 = case shown="\"Disconnect from package\"" w951 {
                  selector: w951 -> [w962 _ w987 _ _]
                  tunnel: w950 -> [w964 w984 w991 w1023 w1032]
                  tunnel: w949 -> [w957 w982 w986 w1021 w1034]
                  tunnel: [w959 w981 w985 w1020 w1031] -> w953
                  tunnel: w952 -> [w963 _ _ w1016 _]
                  tunnel: [w958 w984 w991 w1022 w1032] -> w954
                  tunnel: w948 -> [w955 _ _ w1019 _]
                  tunnel: w947 -> [_ _ _ w1018 _]
                  tunnel: w946 -> [_ _ _ w1017 _]
                  frame Default {
                    n320 = call-dynamic "ExecuteMenuCommand.vi"("reference"=w963, "Command"=w962, "error in (no error)"=w964) -> ("EditorAction"=w961:T45, "FlattenCommandSettings"=w960:T15, "error out"=w956:errorcluster)  [unwired: 13 in, 1 out]
                    n321 = case shown="\"ExecuteCommand\"" w961 {
                      tunnel: w957 -> [w965 w969 w980]
                      tunnel: [w965 w970 w976] -> w959
                      tunnel: w960 -> [_ _ w978]
                      tunnel: w956 -> [w966 w974 w977]
                      tunnel: [w966 w972 w977] -> w958
                      tunnel: w955 -> [_ w967 _]
                      frame "NoAction", Default {
                      }
                      frame "Repaint" {
                        n322 = call-dynamic "layout.vi"("reference"=w967, "error in (no error)"=w974) -> ("error out"=w973:errorcluster)  [unwired: 16 in, 1 out]
                        n323 = Bundle By Name(cluster=w969, "state"=UMLEditor_statesType."Repaint") -> (w968:T7)
                        n324 = call <resource>:"UMLEditor setDiagramInfo.vi"("error in (no error)"=w973, "localVariablesIn"=w968, "action"=enum16{"Name/Dir", "Unsaved", "Saved"}."Unsaved") -> ("localVariablesOut"=w970:T7, "error out"=w972:errorcluster)  [unwired: 2 in, 13 out]
                      }
                      frame "ExecuteCommand" {
                        n325 = Bundle By Name(cluster=w980, "state"=UMLEditor_statesType."ExecuteCommand", "FlattenCommandSettings"=w978) -> (w976:T7)
                      }
                    }
                  }
                  frame "Apply Design Pattern..." {
                    n326 = Bundle By Name(cluster=w982, "state"=UMLEditor_statesType."ApplyDesignPattern") -> (w981:T7)
                  }
                  frame "Remove Node", "Remove package only" {
                    n327 = Equal?(x=w987, y="Remove package only") -> (x = y?=w988:bool)
                    n328 = Bundle By Name(cluster=w986, "state"=UMLEditor_statesType."RemoveSelected", "Don'tDeleteChildren"=w988) -> (w985:T7)
                  }
                  frame "Disconnect from package" {
                    n329 = call-dynamic "GetParentsRecurivly.vi"("reference"=w1016, "error in (no error)"=w1023) -> ("Parents"=w994:refnum<class "AbstractNode.lvclass">[], "error out"=w996:errorcluster)  [unwired: 15 in, 1 out]
                    n330 = Index Array(array=w994) -> (element=w993:refnum<class "AbstractNode.lvclass">)  [unwired: 1 in]
                    n331 = call-dynamic "removeChild.vi"("reference"=w993, "node"=w1016, "error in (no error)"=w996) -> ("reference out"=w1009:refnum<class "AbstractNode.lvclass">, "error out"=w1012:errorcluster)  [unwired: 15 in]
                    n332 = call-dynamic "setParent.vi"("reference"=w1016, "node"=refnum<class "AbstractNode.lvclass"> refnum, "error in (no error)"=w1012) -> ("error out"=w1010:errorcluster)  [unwired: 15 in, 1 out]
                    n333 = call-dynamic "layout.vi"("reference"=w1009, "graph"=w1019, "graphics"=w1018, "grid"=w1017, "error in (no error)"=w1010) -> ("error out"=w1008:errorcluster)  [unwired: 13 in, 1 out]
                    n334 = Delete From Array(array=w994) -> (deleted portion=w995:refnum<class "AbstractNode.lvclass">)  [unwired: 2 in, 1 out]
                    n335 = call-dynamic "getBounds.vi"("reference"=w995, "error in (no error)"=w1008) -> ("bounds"=w1006:T13, "error out"=w1007:errorcluster)  [unwired: 15 in, 1 out]
                    n336 = call <resource>:"Rectangel GetRectInfo.vi"("bounds"=w1006) -> ("maxX"=w1004:dbl)  [unwired: 1 in, 17 out]
                    n337 = call-dynamic "getBounds.vi"("reference"=w1016, "error in (no error)"=w1007) -> ("reference out"=w999:refnum<class "AbstractNode.lvclass">, "bounds"=w1005:T13, "error out"=w998:errorcluster)  [unwired: 15 in]
                    n338 = Unbundle By Name(w1005) -> ("x"=w1003:dbl)
                    n339 = Subtract(x=w1004, y=w1003) -> (x-y=w1002:dbl)
                    n340 = Add(x=10.0, y=w1002) -> (x+y=w1000:dbl)
                    n341 = Greater Or Equal To 0?(x=w1000) -> (x >= 0?=w997:bool)
                    n342 = case shown="True" w997 {
                      tunnel: [w1025 w1030] -> w1015
                      tunnel: w1000 -> [_ w1029]
                      tunnel: w999 -> [_ w1028]
                      tunnel: w998 -> [w1025 w1027]
                      frame False {
                      }
                      frame True {
                        n343 = call-dynamic "translate.vi"("reference"=w1028, "dx"=w1029, "dy"=0.0, "error in (no error)"=w1027) -> ("error out"=w1030:errorcluster)  [unwired: 14 in, 1 out]
                      }
                    }
                    n344 = Bundle By Name(cluster=w1021, "state"=UMLEditor_statesType."Repaint") -> (w992:T7)
                    n345 = call-dynamic "layout.vi"("reference"=w1019, "error in (no error)"=w1015) -> ("error out"=w1013:errorcluster)  [unwired: 16 in, 1 out]
                    n346 = call <resource>:"UMLEditor setDiagramInfo.vi"("error in (no error)"=w1013, "localVariablesIn"=w992, "action"=enum16{"Name/Dir", "Unsaved", "Saved"}."Unsaved") -> ("localVariablesOut"=w1020:T7, "error out"=w1022:errorcluster)  [unwired: 2 in, 13 out]
                  }
                  frame "Configure Node" {
                    n347 = Bundle By Name(cluster=w1034, "state"=UMLEditor_statesType."EditSelected") -> (w1031:T7)
                  }
                }
              }
            }
          }
          event "PictureMenuEvent": Value Change {
            n348 = event-data() -> ("NewVal"=w1035:string)  [unwired: 1 out]
            n349 = Unbundle By Name(w1039) -> ("selcted"=w1043:T9, "selectedEdge"=w1037:refnum<class "AbstractEdge.lvclass">, "SelectedNodes"=w1041:refnum<class "AbstractNode.lvclass">[])
